vi "Read Data.vi"(8 "error in":errorcluster, 11 "CutomOOB_Rx in":refnum<class "TemplateOOB_Rx.lvclass">) -> (0 "error out":errorcluster, 2 "Data":T1, 3 "CutomOOB_Rx out":refnum<class "TemplateOOB_Rx.lvclass">)   [LabVIEW 2021, in "TemplateOOB_Rx.lvclass"]
uses:
  TemplateOOB_Rx.lvclass
  C:/Program Files/National Instruments/LabVIEW 2021/vi.lib/CIF Foundation/CIF Out of Band Commands/CIFOutOfBand.lvclass
  Typedef/gRPC to Main Command Data.ctl
  <vilib>/CIF Foundation/CIF Out of Band Commands/CIFOutOfBand.lvclass/CIFOutOfBand.ctl
  <vilib>/CIF Foundation/CIF Out of Band Commands/Accessors/Read Local OOB Data.vi
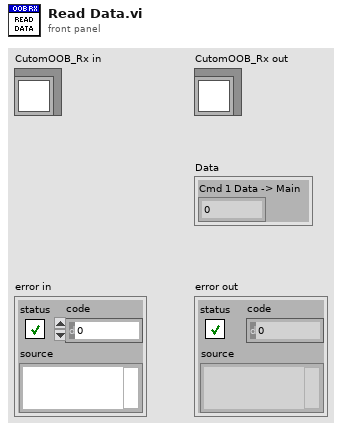
[diagram p1: front panel]
types:
  T1 = typedef "TemplateOOB_Rx.lvclass/gRPC to Main Command Data.ctl" = cluster{"Cmd 1 Data -> Main":i32}
  T2 = typedef "TemplateOOB_Rx.lvclass/Payload.ctl" = cluster{"Data":T1}
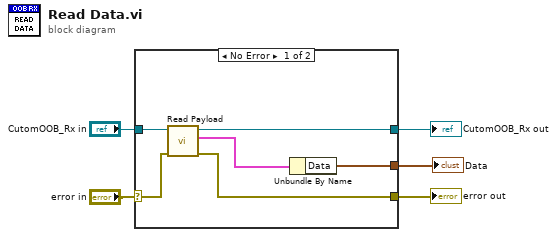
[diagram p0: block diagram]
diagram:
  n1 = case shown="No Error" "error in" {
    selector: "error in" -> [w9 w13]
    tunnel: [w8 w13] -> w5
    tunnel: [w10 w12] -> w4
    tunnel: "CutomOOB_Rx in" -> [w11 w12]
    tunnel: [w6 _] -> w1
    frame No Error {
      n2 = call "Read Payload.vi"("error in"=w9, "CutomOOB_Rx in"=w11) -> ("error out"=w8:errorcluster, "data"=w7:T2, "CutomOOB_Rx out"=w10:refnum<class "TemplateOOB_Rx.lvclass">)  [unwired: 7 in]
      n3 = Unbundle By Name(w7) -> ("Data"=w6:T1)
    }
    frame Error {
    }
  }
  "error out" <- w5
  "CutomOOB_Rx out" <- w4
  "Data" <- w1
